vi "interp_2d.vi"(4 "Scale":sgl[](array[numeric]), 6 "Offset":sgl[](array[numeric]), 8 "Input x":sgl[](array[numeric]), 10 "Set LUT":bool, 11 "Table":sgl[][][](array[numeric])) -> (2 "Output f(x)":sgl[](array[numeric]) format="%#.2f")   [LabVIEW 2013]
panel:
  # "To avoid copying of LUT, call once with \"Set LUT\" true, and false thereafter.  This caches the Table , Scale and Offset, which then need not be passed again.  This differs from interp_4D in that it is reentrant, allowing you to have more than one table, but requiring each call site to be initialized separately. \n\nWarning: This routine uses the first X vector component to index the first LUT dimension, and so on (the same as interp_4d).  This will get you in trouble if you think of Y going vertically and X going horizontally in the 2D table display (Matlab meshgrid style.)  Transpose the LUT if necessary.  This isn't really a row-major/column-major issue.  In matlab you have to say lut(y_ix, x_ix) too.  They just do it that way so it prints out nice."
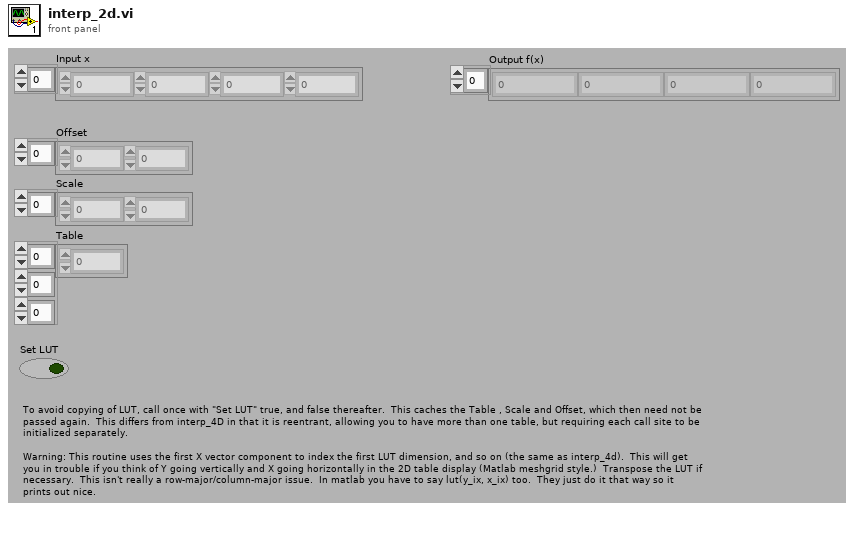
[diagram p1: front panel]
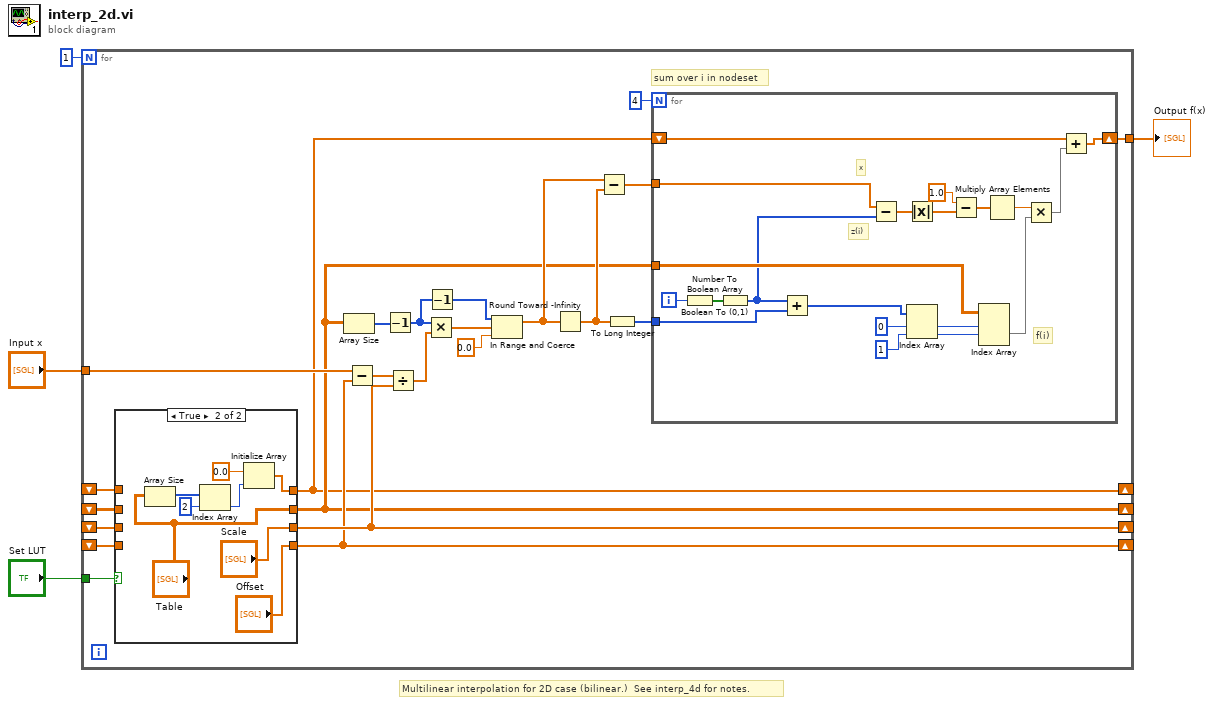
[diagram p0: block diagram]
diagram:
  # "Multilinear interpolation for 2D case (bilinear.)  See interp_4d for notes."
  n1 = for {
    N: 1 -> [_]
    tunnel: "Input x" -> [w21]
    shift-right: [w7] -> _
    shift-left: _ -> [w8]
    shift-right: [w14] -> _
    shift-left: _ -> [w11]
    shift-right: [w13] -> _
    shift-left: _ -> [w10]
    tunnel: "Set LUT" -> [w12]
    tunnel: [w9] -> w2
    shift-right: [w5] -> _
    shift-left: _ -> [w6]
    # "sum over i in nodeset"
    n2 = case shown="True" w12 {
      tunnel: [w31 "Table"] -> w7
      tunnel: [w30 "Scale"] -> w14
      tunnel: [w29 "Offset"] -> w13
      tunnel: w8 -> [w31 _]
      tunnel: w11 -> [w30 _]
      tunnel: w10 -> [w29 _]
      tunnel: [w28 w35] -> w5
      tunnel: w6 -> [w28 _]
      frame False {
      }
      frame True {
        n3 = Array Size(array="Table") -> (size(s)=w39:i32[])
        n4 = Index Array(array=w39, index=2) -> (element=w37:i32)
        n5 = Initialize Array(sgl 0.0, w37) -> (w35:sgl[])
      }
    }
    n6 = Array Size(array=w7) -> (size(s)=w24:i32[])
    n7 = Subtract(x=w21, y=w13) -> (x-y=w22:sgl[])
    n8 = Decrement(x=w24) -> (x-1=w16:i32[])
    n9 = Divide(x=w22, y=w14) -> (x/y=w19:sgl[])
    n10 = Multiply(x=w16, y=w19) -> (x*y=w17:sgl[])
    n11 = Decrement(x=w16) -> (x-1=w15:i32[])
    n12 = In Range and Coerce(upper limit=w15, x=w17, lower limit=sgl 0.0) -> (coerced(x)=w18:sgl[])  [unwired: 1 out]
    n13 = Round Toward -Infinity(1:w18) -> (0:w25:sgl[])
    n14 = Subtract(x=w18, y=w25) -> (x-y=w26:sgl[])
    n15 = To Long Integer(number=w25) -> (32bit integer=w27:i32[])
    n16 = for {
      N: 4 -> [_]
      tunnel: w27 -> [w42]
      tunnel: w7 -> [w56]
      shift-right: [w40] -> w9
      shift-left: w5 -> [w46]
      tunnel: w26 -> [w41]
      i -> [w45]
      # "x"
      # "z(i)"
      # "f(i)"
      n17 = Number To Boolean Array(number=w45) -> (Boolean array=w59:bool[])
      n18 = Boolean To (0,1)(Boolean=w59) -> (0, 1=w44:i16[])
      n19 = Add(x=w44, y=w42) -> (x+y=w43:i32[])
      n20 = Subtract(x=w41, y=w44) -> (x-y=w53:sgl[])
      n21 = Absolute Value(x=w53) -> (abs(x)=w52:sgl[])
      n22 = Index Array(array=w43, index #1=0 ("index"), index #2=1 ("index")) -> (element #1=w55:i32, element #2=w54:i32)
      n23 = Subtract(x=sgl 1.0, y=w52) -> (x-y=w50:sgl[])
      n24 = Index Array(array=w56, index (dim 0)=w55, index (dim 1)=w54) -> (element=w48:sgl[])  [unwired: 1 in]
      n25 = Multiply Array Elements(1:w50) -> (0:w49:sgl)
      n26 = Multiply(x=w49, y=w48) -> (x*y=w47:sgl[])
      n27 = Add(x=w46, y=w47) -> (x+y=w40:sgl[])
    }
  }
  "Output f(x)" <- w2
